vi "Get Version.vi"(8 "error in (no error)":errorcluster) -> (0 "error out":errorcluster, 1 "Path to Exe":path, 3 "Version":string)   [LabVIEW 2014]
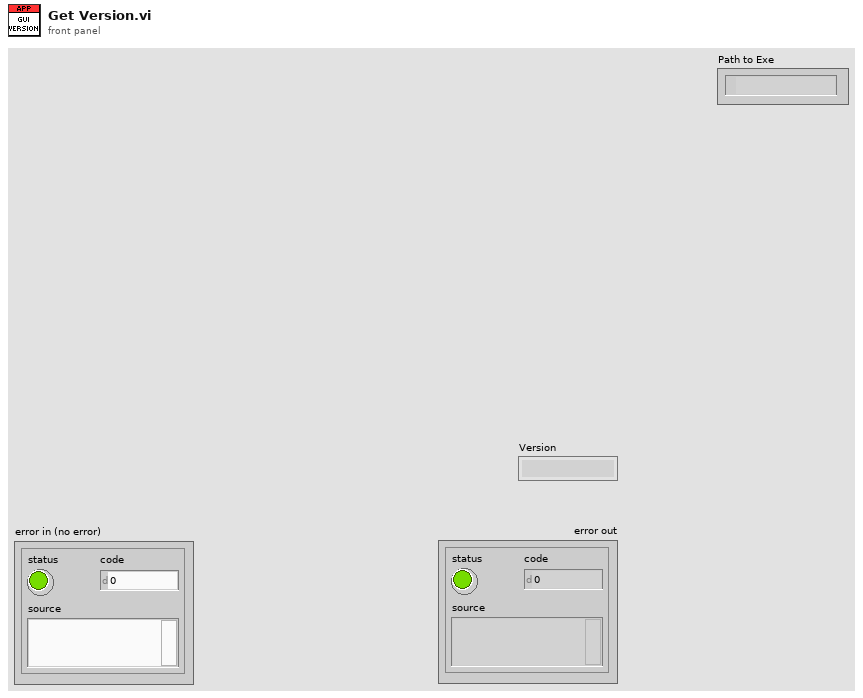
[diagram p1: front panel]
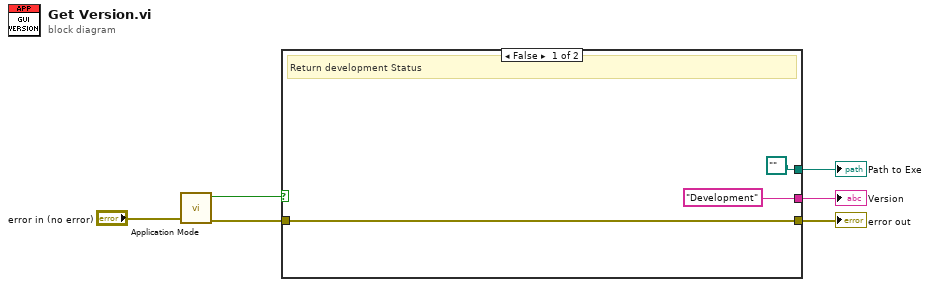
[diagram p0: block diagram]
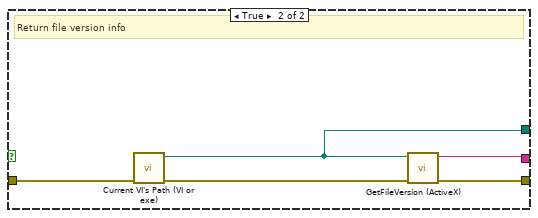
[diagram p2: hidden frame]
diagram:
  n1 = call "Application Mode.vi"("error in (no error)"="error in (no error)") -> ("error out"=w4:errorcluster, "Run Time Mode?"=w5:bool)  [unwired: 9 in]
  n2 = case shown="False" w5 {
    tunnel: ["Development" ("FileVersion") w13] -> w6
    tunnel: w4 -> [w9 w11]
    tunnel: [w9 w14] -> w1
    tunnel: [path "" ("Full Path to VI or executable") w10] -> w2
    frame False {
      # "Return development Status"
    }
    frame True {
      # "Return file version info"
      n3 = call "Current VI's Path (VI or exe).vi"("Error In"=w11) -> ("Error Out"=w12:errorcluster, "VI or executable installation directory"=w10:path)  [unwired: 9 in]
      n4 = call "GetFileVersion (ActiveX).vi"("error in (no error)"=w12, "Filespec"=w10) -> ("error out"=w14:errorcluster, "Full version"=w13:string)  [unwired: 6 in, 2 out]
    }
  }
  "Version" <- w6
  "error out" <- w1
  "Path to Exe" <- w2
